vi "Alter the IP Address of a protocol.vi"(8 "error in (no error)":errorcluster, 10 "IP Address":string, 11 "instrument addon refnum in":T1 format="%.0x") -> (0 "error out":errorcluster, 3 "instrument addon refnum out":T1=18446744073709551615 format="%.0x")   [LabVIEW 2018]
uses:
  <vilib>/NI Veristand/Custom Device API/Custom Device Item Ref.ctl
  <vilib>/addons/VeriStand Custom Device Scripting APIs/Instrument Addon/Libraries Directory/Protocols.lvlibp/TCP/TCP Settings.ctl
  <vilib>/addons/VeriStand Custom Device Scripting APIs/Instrument Addon/API/Custom Device/TCP Factory.vi
  <vilib>/addons/VeriStand Custom Device Scripting APIs/Instrument Addon/API/Custom Device/AK TCP Factory.vi
  <vilib>/addons/VeriStand Custom Device Scripting APIs/Instrument Addon/API/Instrument Addon Scripting API.lvlib
  <vilib>/addons/VeriStand Custom Device Scripting APIs/Instrument Addon/Libraries Directory/Protocols.lvlibp/TCP/TCP.lvclass
  <vilib>/NI Veristand/Custom Device API/Custom Device API.lvlib
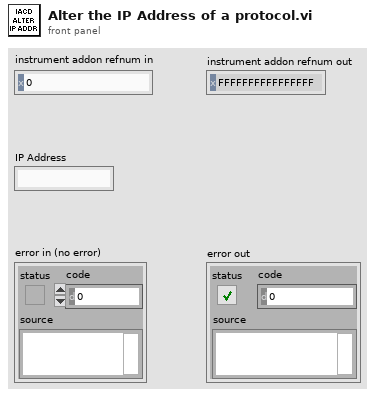
[diagram p1: front panel]
types:
  T1 = typedef "Custom Device API.lvlib/Custom Device Item Ref.ctl" = u64
  T2 = typedef "Protocols.lvlibp/TCP.lvclass/TCP Settings.ctl" = cluster{"IP Address":string, "Port":u16}
  T3 = typedef "Protocols.lvlibp/Protocol Parent.lvclass/Protocol Type.ctl" = enum16{"RS-XXX", "AK RS-XXX", "VISA", "TCPIP", "AK TCPIP", "UDP", "GPIB ConvBox"}
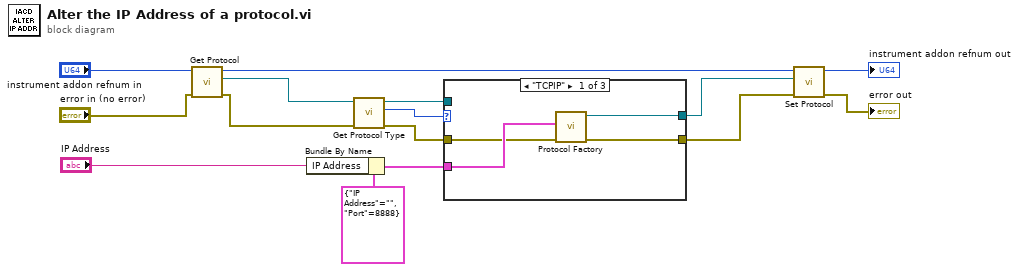
[diagram p0: block diagram]
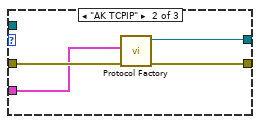
[diagram p2: hidden frame]
diagram:
  n1 = call <vilib>:"Get Protocol.vi"("error in (no error)"="error in (no error)", "instrument addon refnum in"="instrument addon refnum in") -> ("error out"=w10:errorcluster, "protocol"=w12:refnum<class "Protocol Parent.lvclass">, "instrument addon refnum out"=w3:T1)  [unwired: 7 in]
  n2 = Bundle By Name(cluster=T2 {"IP Address"="", "Port"=8888} ("TCP settings"), "IP Address"="IP Address") -> (w7:T2)
  n3 = call <vilib>:"Get Protocol Type.vi"("error in (no error)"=w10, "protocol  in"=w12) -> ("error out"=w6:errorcluster, "protocol type"=w9:T3, "protocol out"=w8:refnum<class "Protocol Parent.lvclass">)  [unwired: 7 in]
  n4 = case shown="\"TCPIP\"" w9 {
    tunnel: w8 -> [_ _ w24]
    tunnel: w7 -> [w19 w20 _]
    tunnel: w6 -> [w18 w21 w25]
    tunnel: [w17 w22 w24] -> w5
    tunnel: [w16 w23 w25] -> w4
    frame "TCPIP" {
      n5 = call-poly <vilib>:"Protocol Factory.vi"("error in (no error)"=w18, "settings"=w19) -> ("error out"=w16:errorcluster, "protocol out"=w17:refnum<class "Protocol Parent.lvclass">)  [unwired: 8 in]
    }
    frame "AK TCPIP" {
      n6 = call-poly <vilib>:"Protocol Factory.vi"("error in (no error)"=w21, "settings"=w20) -> ("error out"=w23:errorcluster, "protocol out"=w22:refnum<class "Protocol Parent.lvclass">)  [unwired: 8 in]
    }
    frame Default {
    }
  }
  n7 = call <vilib>:"Set Protocol.vi"("error in (no error)"=w4, "protocol"=w5, "instrument addon refnum in"=w3) -> ("error out"=→"error out":errorcluster, "instrument addon refnum out"=→"instrument addon refnum out":T1)  [unwired: 7 in]
